vi "AnalyseClassFile.vi"(9 "Overwrite LabVIEW Folder(If empty use this version of LabVIEW)":path, 11 "File Path":path) -> (2 "IsInterface":bool, 3 "ParentLibraries":path[](array[path]))   [LabVIEW 2020, in "DependencyViewer.lvlib"]
uses:
  DependencyViewer/DependencyViewer.lvlib
  <vilib>/regexp/Match Regular Expression.xnode
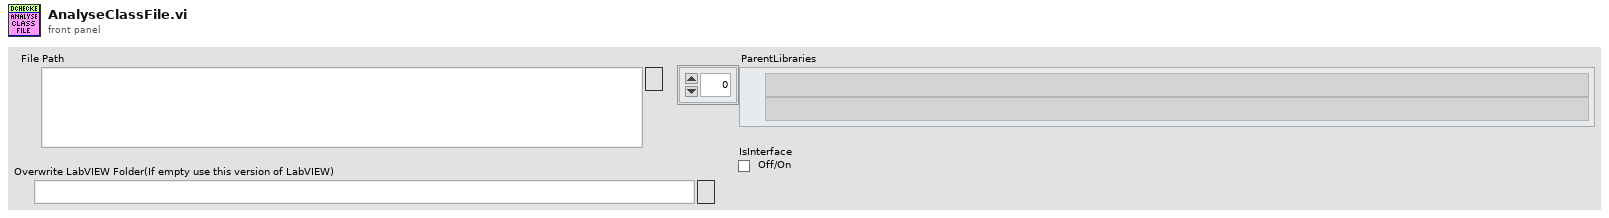
[diagram p1: front panel]
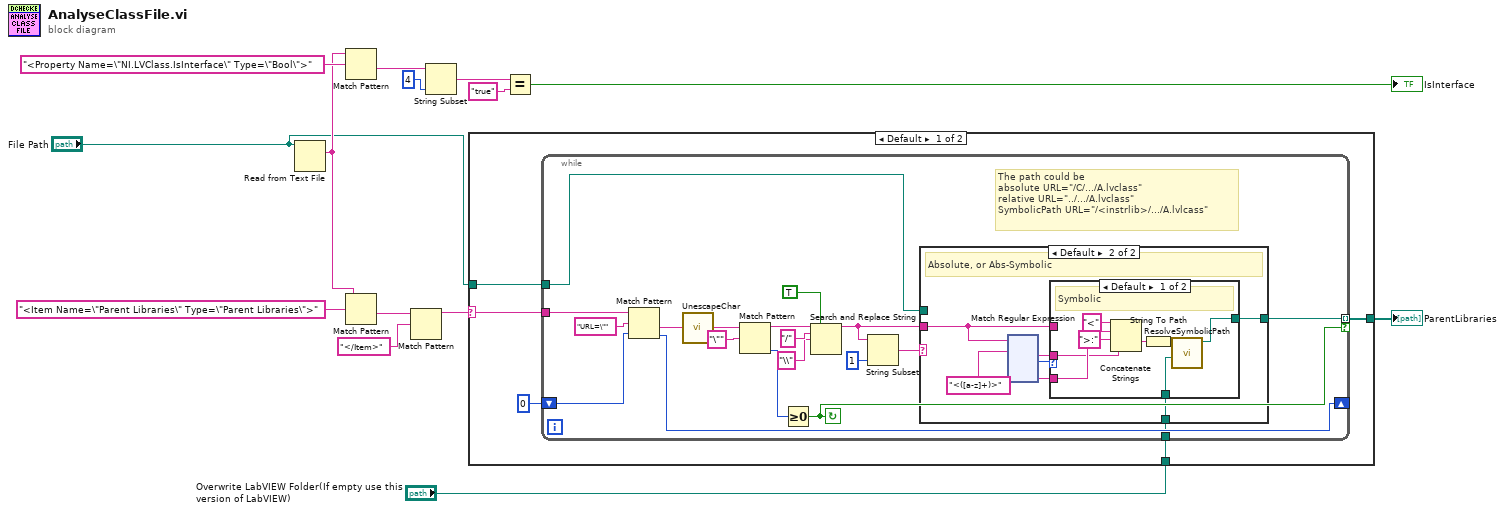
[diagram p0: block diagram]
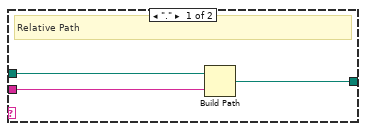
[diagram p2: hidden frame]
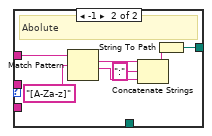
[diagram p3: hidden frame]
diagram:
  n1 = Read from Text File(file (use dialog)="File Path") -> (text=w4:string)  [unwired: 3 in, 3 out]
  n2 = Match Pattern(string=w4, regular expression="<Property Name=\"NI.LVClass.IsInterface\" Type=\"Bool\">") -> (after substring=w13:string)  [unwired: 1 in, 3 out]
  n3 = Match Pattern(string=w4, regular expression="<Item Name=\"Parent Libraries\" Type=\"Parent Libraries\">") -> (after substring=w8:string)  [unwired: 1 in, 3 out]
  n4 = Match Pattern(string=w8, regular expression="</Item>") -> (before substring=w5:string)  [unwired: 1 in, 3 out]
  n5 = String Subset(string=w13, length (rest)=4 ("length (rest)")) -> (substring=w11:string)  [unwired: 1 in]
  n6 = case shown="Default" w5 {
    selector: w5 -> [w19 _]
    tunnel: "File Path" -> [w18 _]
    tunnel: [w17 _] -> w3
    tunnel: "Overwrite LabVIEW Folder(If empty use this version of LabVIEW)" -> [w15 _]
    frame Default {
      n7 = while {
        tunnel: w19 -> [w38]
        tunnel: w18 -> [w22]
        tunnel: [w21] -> w17 mode=indexing if=w34
        shift-right: [w32] -> _
        shift-left: 0 ("offset past match") -> [w33]
        tunnel: w15 -> [w20]
        stop <- w34 continue-if-true
        # "The path could be \nabsolute URL=\"/C/.../A.lvclass\"\nrelative URL=\"../.../A.lvclass\"\nSymbolicPath URL=\"/<instrlib>/.../A.lvlcass\""
        n8 = Match Pattern(string=w38, regular expression="URL=\"", offset (0)=w33) -> (after substring=w27:string, offset past match=w32:i32)  [unwired: 2 out]
        n9 = call <vilib>:"UnescapeChar.vi"("XML In"=w27) -> ("XML Out"=w26:string)  [unwired: 10 in]
        n10 = Match Pattern(string=w26, regular expression="\"") -> (before substring=w31:string, offset past match=w35:i32)  [unwired: 1 in, 2 out]
        n11 = Greater Or Equal To 0?(x=w35) -> (x >= 0?=w34:bool)
        n12 = Search and Replace String(replace all?=TRUE ("replace all? (F)"), input string=w31, search string="/", replace string="\\" ("replace string (\"\")")) -> (result string=w25:string)  [unwired: 4 in, 3 out]
        n13 = String Subset(string=w25, length (rest)=1 ("length (rest)")) -> (substring=w23:string)  [unwired: 1 in]
        n14 = case shown="Default" w23 {
          tunnel: w25 -> [w40 w44]
          tunnel: w22 -> [w41 _]
          tunnel: [w39 w43] -> w21
          tunnel: w20 -> [_ w42]
          frame "." {
            # "Relative Path"
            n15 = Build Path(base path=w41, name or relative path=w40) -> (appended path=w39:path)
          }
          frame Default {
            # "Absolute, or Abs-Symbolic"
            n16 = xnode "Match Regular Expression"("input string"=w44, "regular expression"="<([a-z]+)>") -> ("after match"=w45:string, "offset past match"=w47:i32, "submatch 1"=w46:string)  [unwired: 4 in, 3 out]
            n17 = case shown="Default" w47 {
              tunnel: w44 -> [_ w63]
              tunnel: w46 -> [w56 _]
              tunnel: w45 -> [w54 _]
              tunnel: [w51 w57] -> w43
              tunnel: w42 -> [w50 _]
              frame Default {
                # "Symbolic"
                n18 = Concatenate Strings("<" ("string"), w56, ">:" ("string"), w54) -> (w53:string)
                n19 = String To Path(string=w53) -> (path=w52:path)
                n20 = call "ResolveSymbolicPath.vi"("Overwrite LabVIEW Folder(If empty use this version of LabVIEW)"=w50, "path"=w52) -> ("File Path"=w51:path)  [unwired: 9 in]
              }
              frame -1 {
                # "Abolute"
                n21 = Match Pattern(string=w63, regular expression="[A-Za-z]") -> (match substring=w61:string, after substring=w59:string)  [unwired: 1 in, 2 out]
                n22 = Concatenate Strings(w61, ":" ("string"), w59) -> (w58:string)
                n23 = String To Path(string=w58) -> (path=w57:path)
              }
            }
          }
        }
      }
    }
    frame "" {
    }
  }
  "ParentLibraries" <- w3
  n24 = Equal?(x=w11, y="true") -> (x = y?=→"IsInterface":bool)
